vi "BehaveLights.vi"(8 "error in (no error)":errorcluster, 10 "BehLightIn":T1, 11 "Blink":bool) -> (0 "error out":errorcluster)   [LabVIEW 2014]
doc: "This VI controls teh Tugs three Behavior Lights. Note only one color can be on at a time."
uses:
  <vilib>/myRIO/Express VI/Onboard IO/DO/DO Express VI.xnode
  <vilib>/myRIO/Instrument Drivers/Onboard IO/DIO/vis/Write.vi
  <vilib>/myRIO/Instrument Drivers/Onboard IO/DIO/DIO.lvlib
  <vilib>/myRIO/Common/Instrument Driver Framework/myRIO v1.0/DIO/typedefs/DIO Channels Enum.ctl
  <vilib>/myRIO/Common/Instrument Driver Framework/myRIO v1.0/DIO/typedefs/DIO Channels List.ctl
  <vilib>/myRIO/Common/Instrument Driver Framework/Utilities/typedefs/Generic FPGA Reference.ctl
  <vilib>/myRIO/Common/Instrument Driver Framework/Utilities/typedefs/myRIO v1.0 Reference.ctl
  <vilib>/myRIO/Common/Instrument Driver Framework/Utilities/typedefs/Hardware Version Enum.ctl
  <vilib>/myRIO/Common/Instrument Driver Framework/Utilities/typedefs/myRIO Generic Hardware Reference.ctl
  <vilib>/myRIO/Instrument Drivers/Onboard IO/DIO/typedefs/DIO Reference.ctl
  <vilib>/myRIO/Instrument Drivers/Onboard IO/DIO/vis/myRIO DIO Open.xnode
  <vilib>/myRIO/Common/Instrument Driver Framework/Utilities/vis/Is FPGA Ref Available.vi
  <vilib>/myRIO/Common/Instrument Driver Framework/myRIO v1.0/DIO/vis/myRIO v1.1 Open DIO.vi
  <vilib>/userdefined/High Color/nirio_resource_hc.ctl
panel:
  # "This VI lights up and flashes\nthe robots 3 behavior lights"
  # "Note: Only one color can be on at a time"
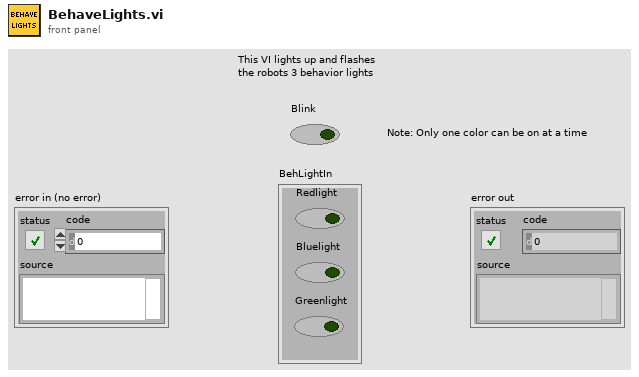
[diagram p1: front panel]
types:
  T1 = cluster{"Redlight":bool, "Bluelight":bool, "Greenlight":bool}
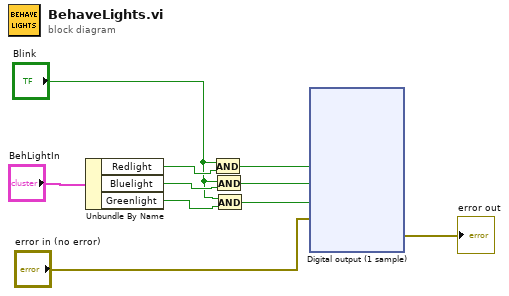
[diagram p0: block diagram]
diagram:
  n1 = Unbundle By Name("BehLightIn") -> ("Redlight"=w9:bool, "Bluelight"=w8:bool, "Greenlight"=w7:bool)
  n2 = And(x="Blink", y=w9) -> (x .and. y?=w3:bool)
  n3 = And(x="Blink", y=w8) -> (x .and. y?=w2:bool)
  n4 = And(x="Blink", y=w7) -> (x .and. y?=w1:bool)
  n5 = xnode ("Digital output (1 sample)")("RedLight (C/DIO0 (DIO0))"=w3, "BlueLight (C/DIO1 (DIO1))"=w2, "Greenlight (C/DIO2 (DIO2))"=w1, "error in (no error)"="error in (no error)") -> ("error out"=→"error out":errorcluster)
